vi "Driver VISA Read with Length.vi"(6 "Timeout":u32=100, 8 "error in (no error)":errorcluster, 9 "Once Length":u32=1024, 10 "All Length":u32=1024, 11 "VISA resource name":refnum<visa-resource-name>) -> (0 "error out":errorcluster, 2 "Receive":string, 3 "VISA resource name out":refnum<visa-resource-name>)   [LabVIEW 2020]
panel:
  out "Left Length":u32
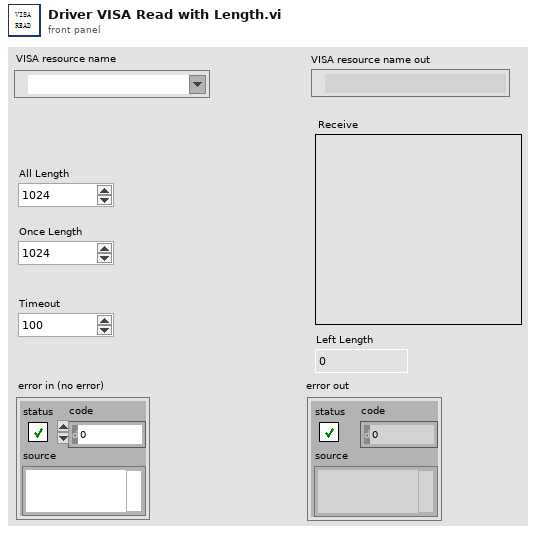
[diagram p1: front panel]
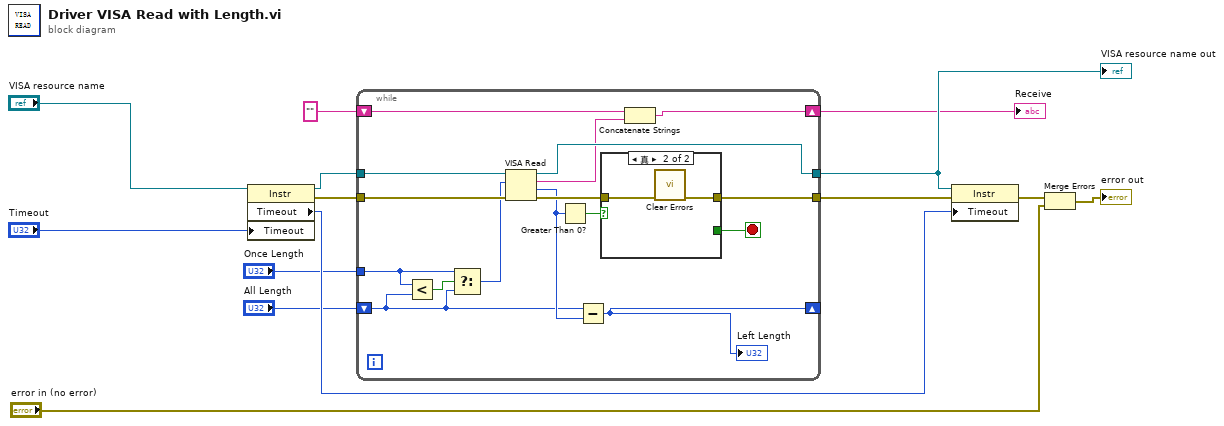
[diagram p0: block diagram]
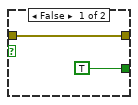
[diagram p2: hidden frame]
diagram:
  n1 = property class="Instr"(reference="VISA resource name", "Timeout"="Timeout") -> (reference out=w7:refnum<visa-resource-name>, error out=w13:errorcluster, "Timeout"=w10:u32)  [unwired: 1 in]
  n2 = while {
    tunnel: w7 -> [w28]
    tunnel: [w29] -> w11
    tunnel: w13 -> [w30]
    tunnel: [w22] -> w9
    shift-right: [w24] -> w3
    shift-left: "" -> [w26]
    tunnel: "Once Length" -> [w17]
    shift-right: [w16] -> _
    shift-left: "All Length" -> [w19]
    stop <- w15 stop-if-true
    n3 = Less?(x=w17, y=w19) -> (x < y?=w20:bool)
    n4 = Select(t=w17, s=w20, f=w19) -> (s? t:f=w18:u32)
    n5 = VISA Read(VISA resource name=w28, byte count=w18, error in (no error)=w30) -> (VISA resource name out=w29:refnum<visa-resource-name>, read buffer=w25:string, return count=w21:u32, error out=w27:errorcluster)
    n6 = Greater Than 0?(x=w21) -> (x > 0?=w23:bool)
    n7 = Subtract(x=w19, y=w21) -> (x-y=w16:u32)
    "Left Length" <- w16
    n8 = case shown="真" w23 {
      tunnel: [w32 w34] -> w22
      tunnel: w27 -> [w32 w33]
      tunnel: [TRUE _] -> w15
      frame False {
      }
      frame True {
        n9 = call <vilib>:"Clear Errors.vi"("error in (no error)"=w33) -> ("error out"=w34:errorcluster)  [unwired: 5 in, 1 out]
      }
    }
    n10 = Concatenate Strings(w26, w25) -> (w24:string)
  }
  "VISA resource name out" <- w11
  "Receive" <- w3
  n11 = property class="Instr"(reference=w11, error in=w9, "Timeout"=w10) -> (error out=w8:errorcluster)  [unwired: 1 out]
  n12 = Merge Errors(w8, "error in (no error)") -> (→"error out":errorcluster)
